vi "2.4.vi"() -> ()   [LabVIEW 2017]
panel:
  out "数值 4":dbl
  in  "数值 3":dbl
  in  "数值 2":dbl
  in  "数值":dbl
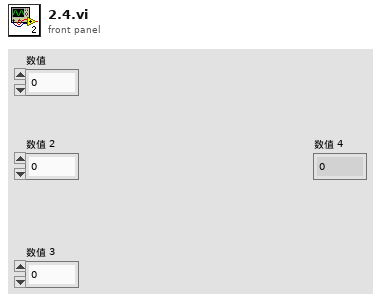
[diagram p1: front panel]
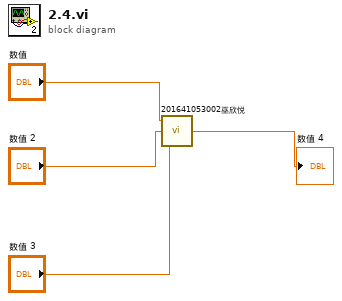
[diagram p0: block diagram]
diagram:
  n1 = call "201641053002巫欣悦.vi"("b"="数值 3", "x"="数值 2", "k"="数值") -> ("y"=→"数值 4":dbl)
